vi "StressFP.vi"(8 "error in (no error)":errorcluster, 10 "Num instructions":i32, 11 "MainQueue":refnum<queue>) -> (0 "error out":errorcluster)   [LabVIEW 2013]
doc: "Stress test for fire pneumatic."
uses:
  QueueInstruction.ctl
  SubsystemEnum.ctl
  ActionEnum.ctl
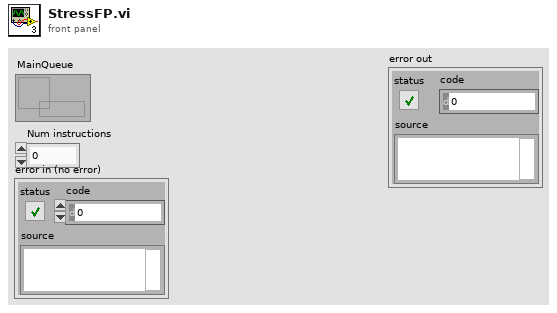
[diagram p1: front panel]
types:
  T1 = typedef "QueueInstruction.ctl" = cluster{"Data":variant, "Subsystem":T2, "Action":T3}
  T2 = typedef "SubsystemEnum.ctl" = enum16{"TankDrive", "FirePneumatic", "Climber", "ClimbWeight", "ShooterAngle"}
  T3 = typedef "ActionEnum.ctl" = enum16{"Init", "SetValue"}
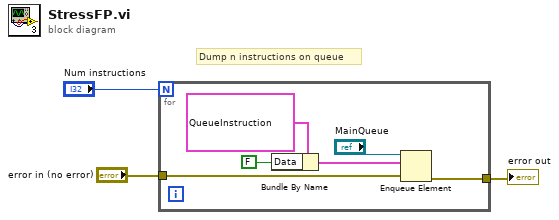
[diagram p0: block diagram]
diagram:
  # "Dump n instructions on queue"
  n1 = for {
    N: "Num instructions" -> [_]
    tunnel: "error in (no error)" -> [w5]
    tunnel: [w4] -> w1
    n2 = Bundle By Name(cluster=T1 {"Data"=variant, "Subsystem"=enum."FirePneumatic", "Action"=enum."SetValue"}, "Data"=FALSE) -> (w6:T1)
    n3 = Enqueue Element(queue="MainQueue", element=w6, error in (no error)=w5) -> (error out=w4:errorcluster)  [unwired: 1 in, 2 out]
  }
  "error out" <- w1
